vi "Format Message String.vi"(0 "Source":string="Error 333 occurred at source of error", 2 "Details":string="reason for problem\nasdfasdf\tasdfaa sdfja ;sldjf;alskdjf;a lksjdf there is way more to this than meets the eye at first glance ;laiwje;fliajsd;flk ajsdlkfja psoieur a;lwdjf; alksjdf;alksdjf; alksedrfap oiwejf;alkw\nwerasdf\t3425 a b c d e f g h i j k l m n o p q\nafsdfasdfasdfasdfas asdf asdf\tasdfasd", 3 "String to Format (not a refnum)":refnum<vi>) -> (1 "message":string="OK", 5 "Bold Start":i32[](array[numeric]), 6 "Bold Length":i32[](array[numeric]), 7 "Source Out":string="Error 333 occurred at source of error", 8 "Details Out":string)   [LabVIEW 2011]
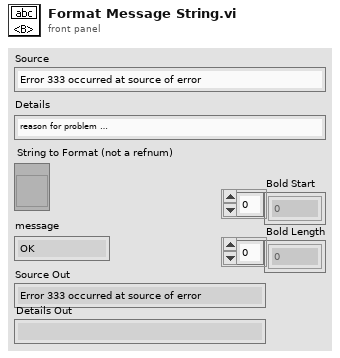
[diagram p1: front panel]
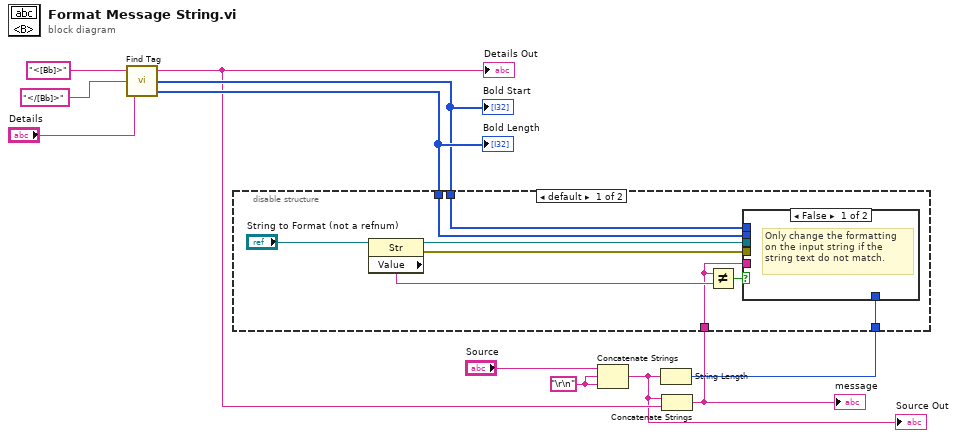
[diagram p0: block diagram]
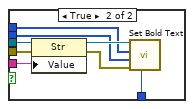
[diagram p2: hidden frame]
diagram:
  w9 = "\r\n"
  n1 = call "Find Tag.vi"("string"="Details", "close tag"="</[Bb]>" ("don't translate!"), "open tag"="<[Bb]>" ("don't translate!")) -> ("Length"=w8:i32[], "Start"=w7:i32[], "string out"=w6:string)
  "Bold Start" <- w7
  "Bold Length" <- w8
  "Details Out" <- w6
  n2 = Concatenate Strings("Source", w9, w9) -> (w3:string)
  "Source Out" <- w3
  n3 = String Length(string=w3) -> (length=w5:i32)
  n4 = Concatenate Strings(w3, w6) -> (w4:string)
  "message" <- w4
  n5 = disable-structure shown="default" {
    disable-tunnel: w8 -> [w20 _]
    disable-tunnel: w7 -> [w19 _]
    disable-tunnel: w5 -> [w13 _]
    disable-tunnel: w4 -> [w12 _]
    frame condition #0 (active) {
      n6 = property class="Str"(reference="String to Format (not a refnum)") -> (reference out=w17:refnum<vi>, error out=w16:errorcluster, "Value"=w15:string)  [unwired: 1 in]
      n7 = Not Equal?(x=w12, y=w15) -> (x != y?=w14:bool)
      n8 = case shown="False" w14 {
        tunnel: w20 -> [_ w26]
        tunnel: w19 -> [_ w25]
        tunnel: w17 -> [_ w24]
        tunnel: w16 -> [_ w23]
        tunnel: w12 -> [_ w22]
        tunnel: w13 -> [_ w21]
        frame False {
          # "Only change the formatting\non the input string if the \nstring text do not match."
        }
        frame True {
          n9 = property class="Str"(reference=w24, error in=w23, "Value"=w22) -> (reference out=w28:refnum<vi>, error out=w27:errorcluster)
          n10 = call "Set Bold Text.vi"("prefix adjustment"=w21, "error in"=w27, "Length"=w26, "Start"=w25, "text"=w28) -> ()  [unwired: 1 in, 1 out]
        }
      }
    }
    frame condition #1 {
      # "Do nothing in RT case."
    }
  }
